vi "FGV User Event Numero.vi"() -> (0 "error out":errorcluster, 3 "User Event Numero":refnum<user-event>)   [LabVIEW 2019]
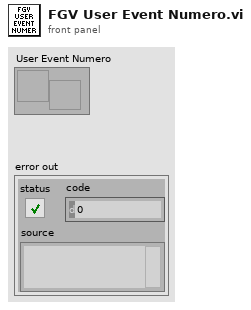
[diagram p1: front panel]
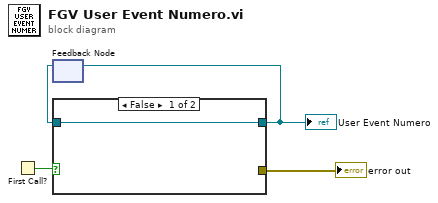
[diagram p0: block diagram]
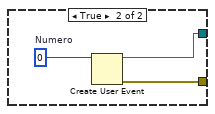
[diagram p2: hidden frame]
diagram:
  n1 = First Call?() -> (First Call?: T/F=w1:bool)
  n2 = feedback #1() -> (w2:refnum<user-event>)  [unwired: 1 in]
  n3 = case shown="False" w1 {
    tunnel: [w5 w7] -> w3
    tunnel: [_ w8] -> w4
    tunnel: w2 -> [w5 _]
    frame False {
    }
    frame True {
      w6 = 0  # Numero
      n4 = Create User Event(user event datatype=w6) -> (user event=w7:refnum<user-event>, error out=w8:errorcluster)  [unwired: 1 in]
    }
  }
  "User Event Numero" <- w3
  "error out" <- w4
  n5 = feedback-in #1(w3) -> ()
